vi "_script_update_template_doc.vi"   [LabVIEW 2014]
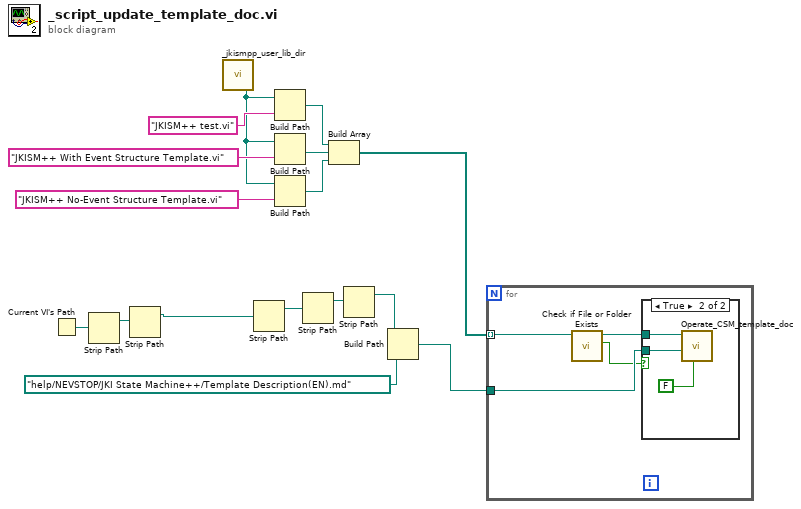
[diagram p0: block diagram]
diagram:
  n1 = Current VI's Path() -> (path=w16:path)
  n2 = Strip Path(path=w16) -> (stripped path=w15:path)  [unwired: 1 out]
  n3 = Strip Path(path=w15) -> (stripped path=w10:path)  [unwired: 1 out]
  n4 = call "_jkismpp_user_lib_dir.vi"() -> ("jkismpp_user.lib_dir"=w2:path)  [unwired: 2 in, 1 out]
  n5 = Strip Path(path=w10) -> (stripped path=w13:path)  [unwired: 1 out]
  n6 = Build Path(base path=w2, name or relative path="JKISM++ test.vi") -> (appended path=w1:path)
  n7 = Build Path(base path=w2, name or relative path="JKISM++ With Event Structure Template.vi") -> (appended path=w7:path)
  n8 = Build Path(base path=w2, name or relative path="JKISM++ No-Event Structure Template.vi") -> (appended path=w6:path)
  n9 = Strip Path(path=w13) -> (stripped path=w14:path)  [unwired: 1 out]
  n10 = Build Array(w1, w7, w6) -> (w5:path[])
  n11 = Strip Path(path=w14) -> (stripped path=w11:path)  [unwired: 1 out]
  n12 = Build Path(base path=w11, name or relative path=path "help/NEVSTOP/JKI State Machine++/Template Description(EN).md" ("Path")) -> (appended path=w4:path)
  n13 = for {
    tunnel: w5 -> [w20] mode=indexing
    tunnel: w4 -> [w19]
    n14 = call <vilib>:"Check if File or Folder Exists.vi"("path"=w20) -> ("file or folder exists?"=w17:bool, "dup path"=w18:path)  [unwired: 8 in, 1 out]
    n15 = case shown="True" w17 {
      tunnel: w19 -> [_ w23]
      tunnel: w18 -> [_ w21]
      frame False {
      }
      frame True {
        n16 = call "Operate_CSM_template_doc.vi"("Save to md(F)/Load to vi(T)"=FALSE, "Path"=w23, "vi path"=w21) -> ()  [unwired: 9 in]
      }
    }
  }
